vi "LSL stream Info.vi"() -> ()   [LabVIEW 2016]
uses:
  lsl.dll
panel:
  out "error out":errorcluster
  in  "source_id":string
  in  "sampling rate":dbl=250.0
  in  "channel_count":i32=1
  in  "type":string="EEG"
  in  "name":string="SS EEG Device"
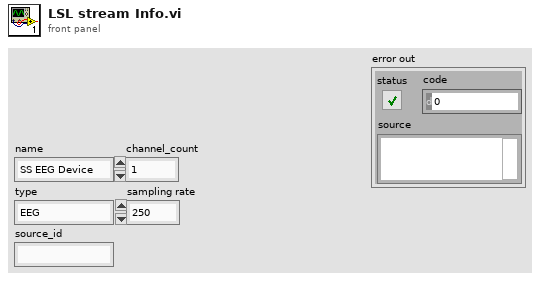
[diagram p1: front panel]
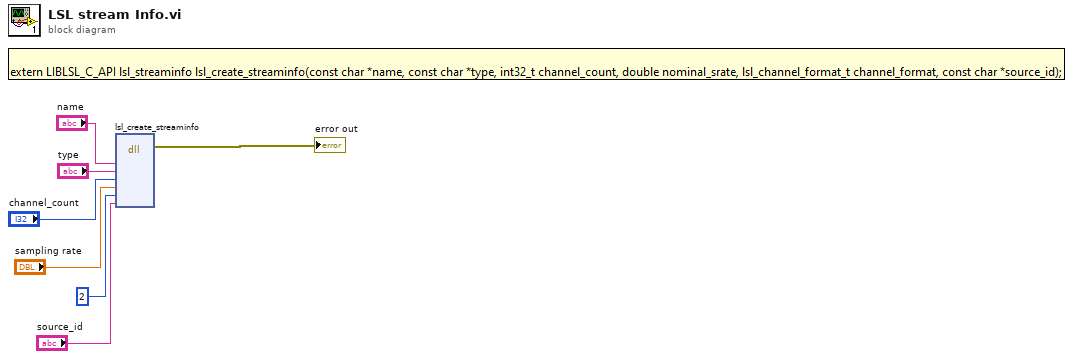
[diagram p0: block diagram]
diagram:
  n1 = dll-call lib="E:/Github Repos/WiBCI16T_Application/Test VI's/lsl.dll" fn="lsl_create_streaminfo"("name"="name", "type"="type", "channel_count"="channel_count", "nominal_state"="sampling rate", "channel_format"=u32 2, "source_id"="source_id") -> (error out=→"error out":errorcluster)  [unwired: 10 in, 1 out]
